vi "Length.vi"(8 "error in (no error)":errorcluster, 11 "Vec3d Class in":refnum<class "Vec3d Class.lvclass">) -> (0 "error out":errorcluster, 2 "Length":dbl, 3 "Vec3d Class out":refnum<class "Vec3d Class.lvclass">)   [LabVIEW 2011, in "Vec3d Class.lvclass"]
uses:
  Vec3d Class.lvclass
  Vec3d Class.lvclass/Vec3d Class.ctl
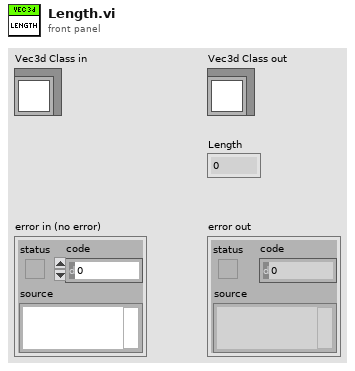
[diagram p1: front panel]
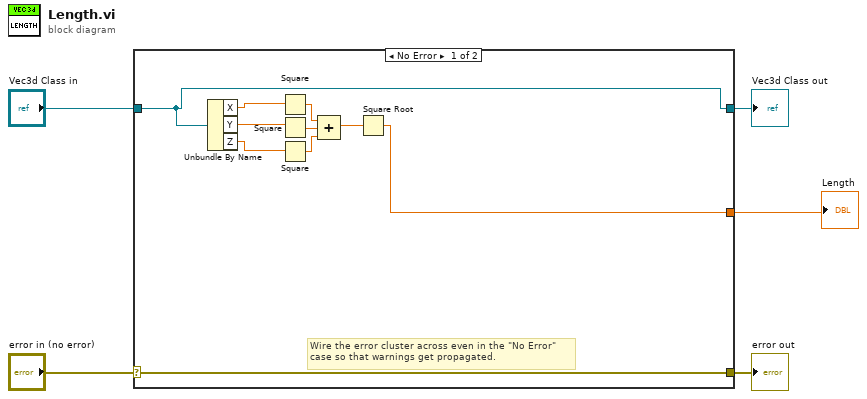
[diagram p0: block diagram]
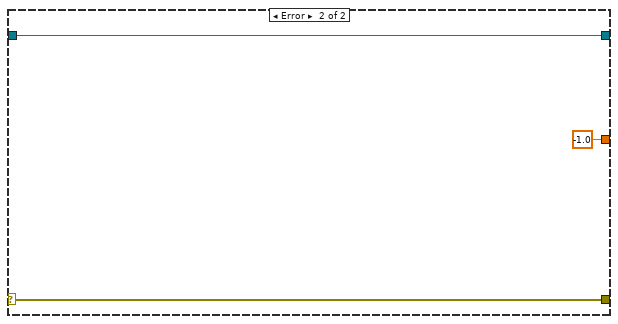
[diagram p2: hidden frame]
diagram:
  n1 = case shown="No Error" "error in (no error)" {
    selector: "error in (no error)" -> [w15 w18]
    tunnel: [w15 w18] -> w4
    tunnel: [w6 w17] -> w2
    tunnel: "Vec3d Class in" -> [w6 w17]
    tunnel: [w7 -1.0] -> w1
    frame No Error {
      # "Wire the error cluster across even in the \"No Error\"\ncase so that warnings get propagated."
      n2 = Unbundle By Name(w6) -> ("X"=w14:dbl, "Y"=w13:dbl, "Z"=w12:dbl)
      n3 = Square(x=w14) -> (x^2=w11:dbl)
      n4 = Square(x=w13) -> (x^2=w10:dbl)
      n5 = Square(x=w12) -> (x^2=w9:dbl)
      n6 = Compound Arithmetic op=ADD(w11, w10, w9) -> (w8:dbl)
      n7 = Square Root(x=w8) -> (sqrt(x)=w7:dbl)
    }
    frame Error {
    }
  }
  "error out" <- w4
  "Vec3d Class out" <- w2
  "Length" <- w1
